vi "FPGA.vi"() -> ()   [LabVIEW 2014]
doc: "This is the primary FPGA VI for the Build Your Own Embedded System project."
uses:
  <vilib>/rvi/Emulation/niFpgaGetClockAttributes.vi
  <vilib>/rvi/Emulation/niFpgaSctlEmulationGetInTimedLoop.vi
  <vilib>/rvi/Emulation/niFpgaEmulationReportErrorSimple.vi
  <vilib>/EmbeddedDisplay/Hitachi HD44780/FPGA/Internal/LCD Command.vi
  <vilib>/EmbeddedDisplay/Hitachi HD44780/FPGA/Public/Command Handler (8 Bits).vi
  <vilib>/rvi/Emulation/niFpgaProcessEmulError.vi
  <vilib>/rvi/Emulation/niFpgaCriticalErrorInLSC.vi
  <vilib>/EmbeddedDisplay/Hitachi HD44780/FPGA/HD44780 FPGA.lvlib
panel:
  in  "LCD Command":T1={"device index (-1)"=-1, "operation (0)"=0}
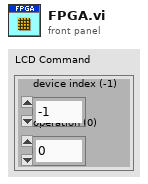
[diagram p1: front panel]
types:
  T1 = cluster{"device index (-1)":i8, "operation (0)":u32}
  T2 = cluster{"RS":refnum<k21>, "R/W":refnum<k21>, "E1":refnum<k21>, "E2":refnum<k21>, "DB0":refnum<k21>, "DB1":refnum<k21>, "DB2":refnum<k21>, "DB3":refnum<k21>, "DB4":refnum<k21>, "DB5":refnum<k21>, "DB6":refnum<k21>, "DB7":refnum<k21>}
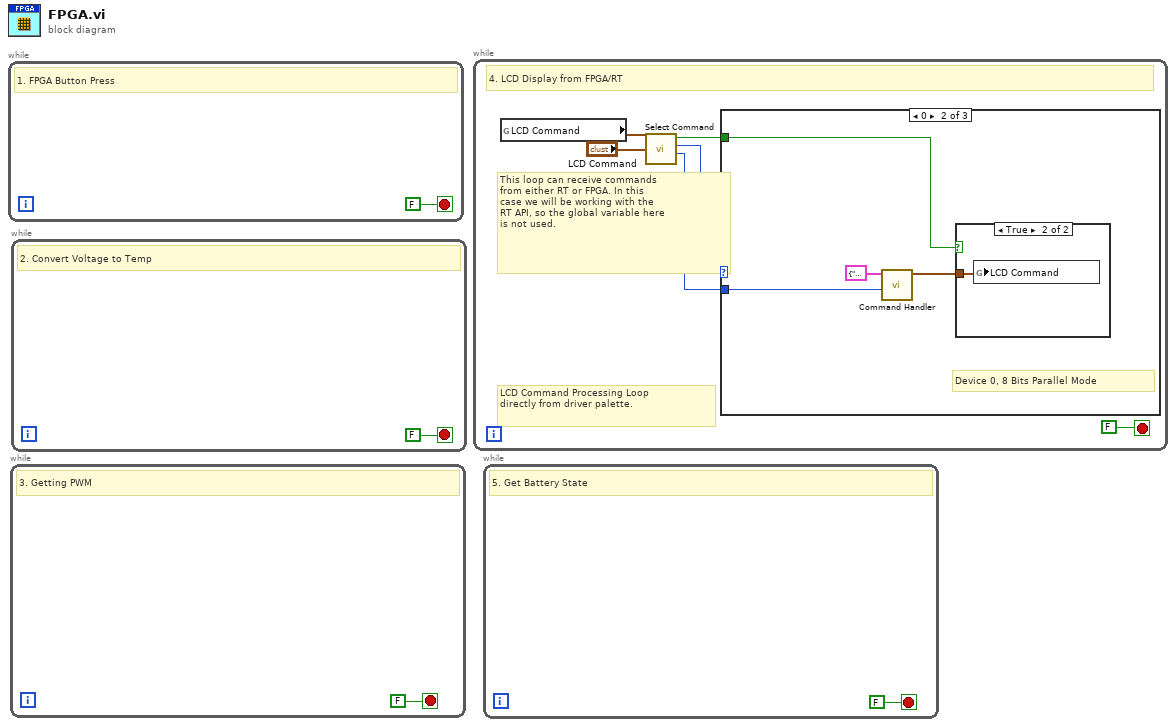
[diagram p0: block diagram]
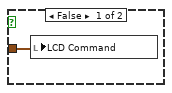
[diagram p3: hidden frame]
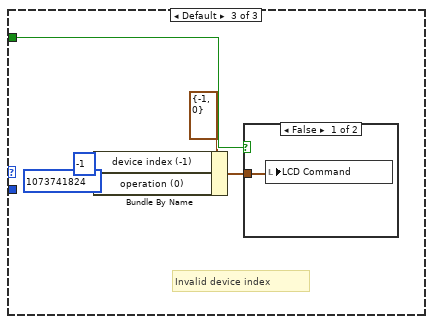
[diagram p4: hidden frame]
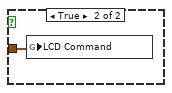
[diagram p5: hidden frame]
diagram:
  n1 = while {
    stop <- FALSE stop-if-true
    # "1. FPGA Button Press"
  }
  n2 = while {
    stop <- FALSE stop-if-true
    # "3. Getting PWM"
  }
  n3 = while {
    stop <- FALSE stop-if-true
    # "2. Convert Voltage to Temp"
  }
  n4 = while {
    stop <- FALSE stop-if-true
    # "4. LCD Display from FPGA/RT"
    # "This loop can receive commands\nfrom either RT or FPGA. In this\ncase we will be working with the \nRT API, so the global variable here\nis not used."
    # "LCD Command Processing Loop\ndirectly from driver palette."
    n5 = global read "LCD Command.vi" "LCD Command"() -> (w4:T1)
    n6 = call <vilib>:"Select Command.vi"("Host LCD Command"="LCD Command", "FPGA LCD Command"=w4) -> ("operation"=w6:u32, "device index"=w7:i8, "FPGA? True : False"=w5:bool)  [unwired: 7 in]
    n7 = case shown="0" w7 {
      tunnel: w6 -> [_ w13 _]
      tunnel: w5 -> [_ w12 w20]
      frame -1 {
        # "IDLE State"
      }
      frame 0 {
        # "Device 0, 8 Bits Parallel Mode"
        n8 = call-poly <vilib>:"Command Handler.vi"("operation"=w13, "device connection map in"=T2 {"RS"="DIO19", "R/W"="DIO18", "E1"="DIO17", "E2"="DIO17", "DB0"="DIO20", "DB1"="DIO21", "DB2"="DIO22", "DB3"="DIO23", "DB4"="DIO24", "DB5"="DIO25", "DB6"="DIO26", "DB7"="DIO27"}) -> ("result"=w11:T1)  [unwired: 9 in]
        n9 = case shown="True" w12 {
          tunnel: w11 -> [w14 w15]
          frame False {
            n10 = local write "LCD Command"(w14) -> ()
          }
          frame True {
            n11 = global write "LCD Command.vi" "LCD Command"(w15) -> ()
          }
        }
      }
      frame Default {
        # "Invalid device index"
        n12 = Bundle By Name(cluster=T1 {"device index (-1)"=-1, "operation (0)"=0} ("LCD Command"), "device index (-1)"=i8 -1 ("LCD_device index (-1)"), "operation (0)"=u32 1073741824 ("LCD_operation (0)")) -> (w16:T1)
        n13 = case shown="False" w20 {
          tunnel: w16 -> [w21 w22]
          frame False {
            n14 = local write "LCD Command"(w21) -> ()
          }
          frame True {
            n15 = global write "LCD Command.vi" "LCD Command"(w22) -> ()
          }
        }
      }
    }
  }
  n16 = while {
    stop <- FALSE stop-if-true
    # "5. Get Battery State"
  }
